vi "balance_query.vi"(8 "error in (no error)":errorcluster, 11 "Database_handler in":refnum<class "Database_handler.lvclass">) -> (0 "error out":errorcluster, 3 "Database_handler out":refnum<class "Database_handler.lvclass">)   [LabVIEW 2025, in "Database_handler.lvlib" / "Database_handler.lvclass"]
uses:
  Database_handler.lvclass
  Database_handler.lvclass/Database_handler.ctl
  DB_fb_tocont Messages/Balance_fb Msg/Balance_fb Msg.lvclass/Balance_fb Msg.ctl
  <vilib>/ActorFramework/Message Enqueuer/Message Enqueuer.lvclass/Message Enqueuer.ctl
  <vilib>/ActorFramework/Message Enqueuer/Enqueue.vi
  DB_fb_tocont Messages/Balance_fb Msg/Balance_fb Msg.lvclass
  <vilib>/ActorFramework/Message Priority Queue/Priority Enqueue.vi
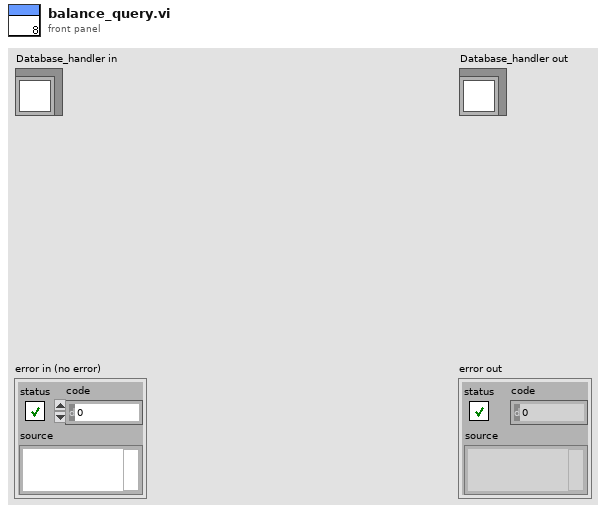
[diagram p1: front panel]
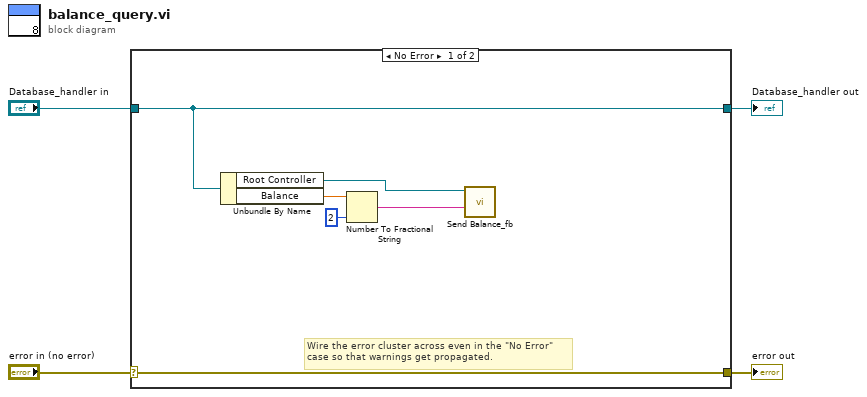
[diagram p0: block diagram]
diagram:
  n1 = case shown="No Error" "error in (no error)" {
    selector: "error in (no error)" -> [w10 w12]
    tunnel: [w10 w12] -> w3
    tunnel: [w6 w11] -> w1
    tunnel: "Database_handler in" -> [w6 w11]
    frame No Error {
      # "Wire the error cluster across even in the \"No Error\"\ncase so that warnings get propagated."
      n2 = Unbundle By Name(w6) -> ("Root Controller"=w5:refnum<class "Message Enqueuer.lvclass">, "Balance"=w9:dbl)
      n3 = Number To Fractional String(number=w9, precision (6)=i16 2) -> (F-format string=w7:string)  [unwired: 2 in]
      n4 = call "Send Balance_fb.vi"("Balance"=w7, "Message Enqueuer"=w5) -> ()  [unwired: 8 in, 2 out]
    }
    frame Error {
    }
  }
  "error out" <- w3
  "Database_handler out" <- w1
